vi "Build Register Message.vi"(0 "Target CSM":string, 5 "Source CSM (* as Default)":string="*", 7 "Status":string, 9 "API (If \"\", Same As \"Status\")":string, 12 "Priority (No Change)":T1) -> (6 "CSM Message String":string)   [LabVIEW 2017, in "Communicable State Machine.lvlib"]
doc: "Concatenates register state operation message strings. The message format is as follows:\n\n //[source-state]@[source-module] >> [response-message]@[response-module] -><register>\n status @ Source >> API @ Target -><register>\n\n Example: Bind the \"Download Finished\" message of the Downloader module to the \"Start Play\" API of the Player module.\n // Bind the \"Download Finished\" message of the Downloader module to the \"Start Play\" API of the Player module\n DownloadFinished@Downloader >> StartPlay@Player -><register>\n // When executing the message within the Player module, \"Player\" can be omitted\n DownloadFinished@Downloader >> StartPlay -><register>\n // When multiple modules have the \"Download Finished\" message,\n // use * to bind this message from all modules to the \"Start Play\" API of the Player module\n DownloadFinished@* >> StartPlay@Player -><register>\n\n\n> [!NOTE] <b>Message Building API</b>\n>\n> This type of API is only used to concatenate message strings and does not send messages directly. The strings need to be merged into the CSM state queue, and the messages will be sent and the operation executed within the Parse State Queue++ VI. If you are familiar with CSM rules, you do not need to use this type of API. You can type the corresponding message string or operation string directly into the string.\n\n\n> [!NOTE] <b>CSM Registration</b>\n>\n> Registration associates a broadcast with a bound interface (API). When the broadcast is triggered, the bound interface (API) is called. Registrations can also be cancelled. In CSM, there are two types of broadcasts:\n>\n> - <b>Broadcast</b>: Broadcast explicitly called by the module sending the broadcast message. Arguments need to be explicitly provided.\n> - <b>State</b>: Any state of a CSM module can also be registered to. The argument received by the triggered API is the Response of the CSM state.\n>\n> // Register\n> [CSM Broadcast]@[SourceModule] >> [Bound API]@[TargetModule] -><register> // [Comments]\n> // Unregister\n> [CSM Broadcast]@[SourceModule] >> [Bound API]@[TargetModule] -><unregister> // [Comments]\n>\n> - <b>CSM Broadcast</b>: Defined by the source module. Refer to \"CSM Broadcast Format Parsing\" for details.\n> - <b>Source Module</b>: The broadcasting module. If registering to broadcasts from any module, the source module can be represented by `*`.\n> - <b>Bound API</b>: Defined by the target module. It is the external interface of the target module.\n> - <b>Target Module</b>: The module where the bound API resides. When indicating registration to the current module within a CSM module, it can be ignored. The preceding `@` separator is also omitted.\n> - `<register>` / `<unregister>`: Definition of the Register/Unregister operation type.\n> - <b>Comments</b>: Comment information, which will not be parsed.\n\n\n> [!NOTE] <b>CSM Registration Location</b>\n>\n> There are two types of registration rules added by CSM registrations: Internal Addition and External Addition.\n> - <b>External Addition</b>: Rules added externally are global rules. They will not be automatically deleted when the CSM module exits and must be manually unregistered.\n> - Rules added using the `-<register>` statement are considered externally added if the module name where the API resides is specified.\n> - All rules added using the API CSM - Register Broadcast VI are considered externally added.\n> - <b>Internal Addition</b>: Rules added internally within a CSM module will be automatically deleted when the CSM module exits, so there is no need to manually unregister.\n> - Rules are considered internally added only when added using the `-<register>` statement and the API does not specify a module name.\n>\n> // Example:\n> status@sourceModule >> API@TargetModule -><register> // Externally added\n> status@sourceModule >> API -><register> // Internally added\n\n\n> [!NOTE] <b>CSM Broadcast Priority</b>\n>\n>Broadcasts have priorities. State broadcast is a special type of broadcast. By default, the priority of state broadcasts is the same as the priority of status broadcasts. Interrupt broadcasts are high-priority broadcasts and are passed using the high-priority queue, just like synchronous messages. Status broadcasts are low-priority broadcasts and are passed using the low-priority queue, just like asynchronous messages.\n>\n> // The default broadcast is a Status Broadcast, for example:\n> ModuleInternalChange >> Arguments -> <broadcast> // Low Priority\n> ModuleInternalChange >> Arguments -> <broadcast> // Low Priority\n>\n> The default priority is defined by the sender via the broadcast type in the broadcast format.\n>\n> // The sender can define the priority of the broadcast\n> ModuleInternalChange >> Arguments -> <status> // Low Priority\n> ModuleInternalChange >> Arguments -> <interrupt> // High Priority\n>\n> Default registrations do not change the priority, but the priority of the registered broadcast can be changed via special registration formats.\n>\n> // Default registration does not change priority\n> ModuleInternalChange@SourceModule >> API@TargetModule -><register>\n> // Change the registered broadcast to Normal priority, regardless of its original priority\n> ModuleInternalChange@SourceModule >> API@TargetModule -><register as status>\n> // Change the registered broadcast to High priority, regardless of its original priority\n> ModuleInternalChange@SourceModule >> API@TargetModule -><register as interrupt>\n\n\n-- <b>Controls</b> --\n- <b>Target CSM</b>: Name of the CSM module registering to the status.\n- <b>Source CSM (* as Default)</b>: Name of the CSM module publishing the status.\n- <b>Status</b>: Status to register.\n- <b>API (If \"\", Same As \"Status\")</b>: Name of the API in the registering module that responds to the status.\n- <b>Priority (No Change)</b>: Priority of the broadcast after registration.\n\n-- <b>Indicators</b> --\n- <b>CSM Message String</b>: Concatenated CSM message string."
uses:
  Communicable State Machine.lvlib
  AdvanceAPI/CSM - Broadcast Message Type.ctl
  _Shared/CSM Shared.lvlib
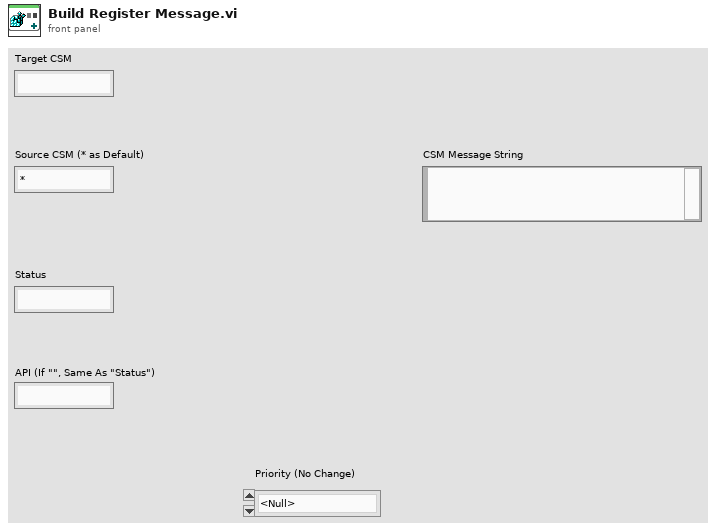
[diagram p1: front panel]
types:
  T1 = typedef "Communicable State Machine.lvlib/CSM - Broadcast Message Type.ctl" = enum16{"<Null>", "Status", "Interrupt"}
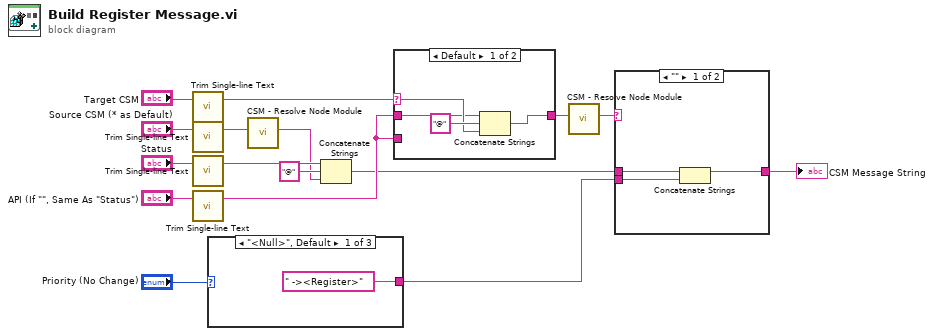
[diagram p0: block diagram]
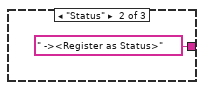
[diagram p2: hidden frame]
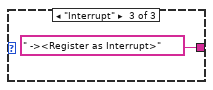
[diagram p3: hidden frame]
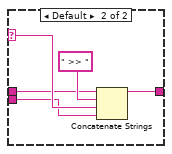
[diagram p4: hidden frame]
diagram:
  n1 = call "Trim Single-line Text.vi"("single-line text"="Target CSM") -> ("trimed text"=w7:string)  [unwired: 2 in]
  n2 = call "Trim Single-line Text.vi"("single-line text"="Source CSM (* as Default)") -> ("trimed text"=w9:string)  [unwired: 2 in]
  n3 = call "Trim Single-line Text.vi"("single-line text"="Status") -> ("trimed text"=w11:string)  [unwired: 2 in]
  n4 = call "Trim Single-line Text.vi"("single-line text"="API (If \"\", Same As \"Status\")") -> ("trimed text"=w8:string)  [unwired: 2 in]
  n5 = case shown="\"<Null>\", Default" "Priority (No Change)" {
    tunnel: [" -><Register>" ("string") " -><Register as Status>" ("string") " -><Register as Interrupt>" ("string")] -> w4
    frame "<Null>", Default {
    }
    frame "Status" {
    }
    frame "Interrupt" {
    }
  }
  n6 = call "CSM - Resolve Node Module.vi"("Node Name"=w9) -> ("CSM Module Name"=w2:string)  [unwired: 10 in]
  n7 = Concatenate Strings(w11, "@" ("string"), w2) -> (w5:string)
  n8 = case shown="Default" w7 {
    selector: w7 -> [w21 _]
    tunnel: [w22 w24] -> w6
    tunnel: w8 -> [w20 w24]
    tunnel: w8 -> [_ _]
    frame Default {
      n9 = Concatenate Strings(w20, "@" ("string"), w21) -> (w22:string)
    }
    frame "" {
    }
  }
  n10 = call "CSM - Resolve Node Module.vi"("Node Name"=w6) -> ("CSM Module Name"=w3:string)  [unwired: 10 in]
  n11 = case shown="\"\"" w3 {
    selector: w3 -> [_ w30]
    tunnel: [w25 w32] -> w16
    tunnel: w5 -> [w27 w29]
    tunnel: w4 -> [w26 w28]
    frame "" {
      n12 = Concatenate Strings(w27, w26) -> (w25:string)
    }
    frame Default {
      n13 = Concatenate Strings(w29, " >> " ("string"), w30, w28) -> (w32:string)
    }
  }
  "CSM Message String" <- w16
